vi "Revision Query.vi"(8 "error in (no error)":errorcluster, 11 "VISA resource name":refnum<visa-resource-name>) -> (0 "error out":errorcluster, 1 "Version Details":string, 2 "Instrument Driver Revision":string, 3 "VISA resource name out":refnum<visa-resource-name>)   [LabVIEW 2021, in "Keithley 2200 Series.lvlib"]
doc: "Queries the current instrument software version and Instrument Driver Revision.\n\nRefer to the Readme file for detailed driver information including modification history."
uses:
  <instrlib>/Keithley 2200 Series/Keithley 2200 Series.lvlib
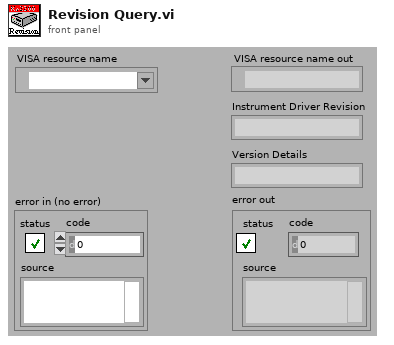
[diagram p1: front panel]
types:
  T1 = enum32{"invalid app kind", "Development System", "Run Time System", "Student Edition", "Embedded LabVIEW", "Evaluation", "Custom"}
  T2 = cluster{"Major":u16, "Minor":u16, "Fix":u16, "Build":u16}
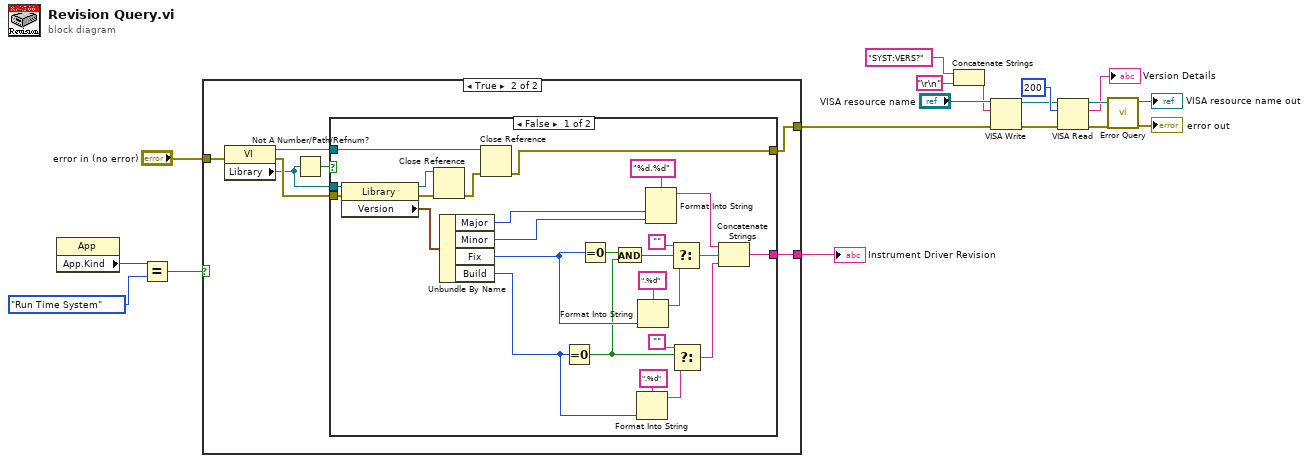
[diagram p0: block diagram]
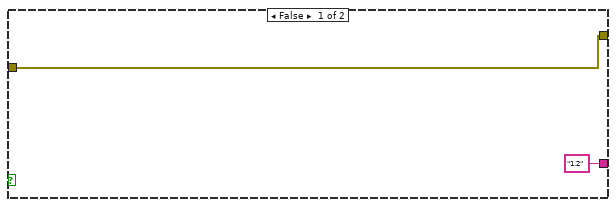
[diagram p2: hidden frame]
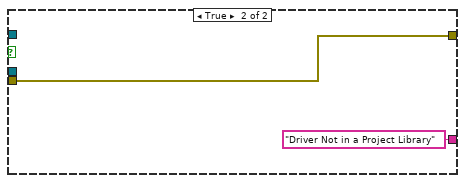
[diagram p3: hidden frame]
diagram:
  n1 = property class="App"() -> ("App.Kind"=w3:T1)  [unwired: 2 in, 2 out]
  n2 = Equal?(x=w3, y=T1."Run Time System" ("Application:Kind")) -> (x = y?=w1:bool)
  n3 = case shown="True" w1 {
    tunnel: ["1.2" w23] -> w6
    tunnel: "error in (no error)" -> [w19 w22]
    tunnel: [w19 w21] -> w4
    frame False {
    }
    frame True {
      n4 = property class="VI"(error in=w22) -> (reference out=w27:refnum<vi>, error out=w26:errorcluster, "Library"=w25:refnum<vi>)  [unwired: 1 in]
      n5 = Not A Number/Path/Refnum?(number/path/refnum=w25) -> (NaN/Path/Refnum?=w24:bool)
      n6 = case shown="False" w24 {
        tunnel: w27 -> [w50 _]
        tunnel: w26 -> [w35 w55]
        tunnel: [w30 w55] -> w21
        tunnel: [w29 "Driver Not in a Project Library"] -> w23
        tunnel: w25 -> [w28 _]
        frame False {
          n7 = property class="Library"(reference=w28, error in=w35) -> (reference out=w52:refnum<vi>, error out=w53:errorcluster, "Version"=w49:T2)
          n8 = Close Reference(reference=w52, error in (no error)=w53) -> (error out=w51:errorcluster)
          n9 = Unbundle By Name(w49) -> ("Major"=w38:u16, "Minor"=w37:u16, "Fix"=w34:u16, "Build"=w36:u16)
          n10 = Close Reference(reference=w50, error in (no error)=w51) -> (error out=w30:errorcluster)
          n11 = Equal To 0?(x=w36) -> (x = 0?=w32:bool)
          n12 = Equal To 0?(x=w34) -> (x = 0?=w33:bool)
          n13 = And(x=w33, y=w32) -> (x .and. y?=w31:bool)
          n14 = Format Into String(format string=".%d", w36) -> (resulting string=w42:string)  [unwired: 2 in, 1 out]
          n15 = Format Into String(format string=".%d", w34) -> (resulting string=w46:string)  [unwired: 2 in, 1 out]
          n16 = Format Into String(format string="%d.%d", w38, w37) -> (resulting string=w44:string)  [unwired: 2 in, 1 out]
          n17 = Select(t="", s=w31, f=w46) -> (s? t:f=w43:string)
          n18 = Select(t="", s=w32, f=w42) -> (s? t:f=w39:string)
          n19 = Concatenate Strings(w44, w43, w39) -> (w29:string)
        }
        frame True {
        }
      }
    }
  }
  "Instrument Driver Revision" <- w6
  n20 = Concatenate Strings("SYST:VERS?" ("write buffer"), "\r\n") -> (w11:string)
  n21 = VISA Write(VISA resource name="VISA resource name", write buffer=w11, error in (no error)=w4) -> (VISA resource name out=w17:refnum<visa-resource-name>, error out=w16:errorcluster)  [unwired: 1 out]
  n22 = VISA Read(VISA resource name=w17, byte count=u32 200 ("byte count(100)"), error in (no error)=w16) -> (VISA resource name out=w14:refnum<visa-resource-name>, read buffer=→"Version Details":string, error out=w13:errorcluster)  [unwired: 1 out]
  n23 = call <instrlib>:"Error Query.vi"("error in (no error)"=w13, "VISA resource name"=w14) -> ("error out"=→"error out":errorcluster, "VISA resource name out"=→"VISA resource name out":refnum<visa-resource-name>)  [unwired: 8 out]
